vi "Check SW Limits.vi"(10 "Dir(Fwd=T)":bool, 11 "Encoder in":i32) -> (3 "Soft Limit?":bool)   [LabVIEW 2015, in "Tool Module.lvlib"]
uses:
  Tool Module.lvlib
  Support/ToolModGLOB.vi
  Tool Config/Tool Cfg.lvlib
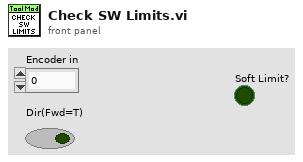
[diagram p1: front panel]
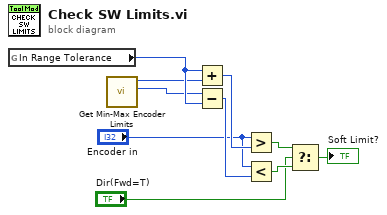
[diagram p0: block diagram]
diagram:
  n1 = global read "ToolModGLOB.vi" "In Range Tolerance"() -> (w10:i32)
  n2 = call "Get Min-Max Encoder Limits.vi"() -> ("MinEncoder"=w8:i32, "MaxEncoder"=w9:i32)  [unwired: 8 in, 2 out]
  n3 = Add(x=w10, y=w9) -> (x+y=w7:i32)
  n4 = Subtract(x=w8, y=w10) -> (x-y=w6:i32)
  n5 = Greater?(x="Encoder in", y=w7) -> (0:w5:bool)
  n6 = Less?(x="Encoder in", y=w6) -> (x < y?=w4:bool)
  n7 = Select(t=w5, s="Dir(Fwd=T)", f=w4) -> (s? t:f=→"Soft Limit?":bool)
